vi "Try Match Response.vi"(8 "error in":errorcluster, 10 "ICAN CC Frame":refnum<class "ICAN CC Frame.lvclass">, 11 "Segmented Upload Transfer":refnum<class "Segmented Upload Transfer.lvclass">) -> (0 "error out":errorcluster, 2 "Match":bool, 3 "SDO Transfer":refnum<class "SDO Transfer.lvclass">)   [LabVIEW 2020, in "CANopen.lvlib" / "SDO Manager.lvlib" / "Segmented Upload Transfer.lvclass"]
uses:
  Segmented Upload Transfer.lvclass
  SDO Transfer/SDO Transfer.lvclass
  HAL/Source/Interfaces/ICAN CC Frame/ICAN CC Frame.lvclass
  Segmented Upload Transfer.lvclass/Segmented Upload Transfer.ctl
  CANopen Message/CANopen Message.lvclass
  SDO Transfer/SDO abort code.ctl
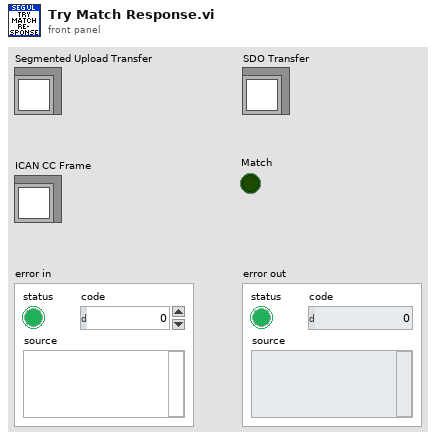
[diagram p1: front panel]
types:
  T1 = typedef "CANopen.lvlib/SDO Manager.lvlib/SDO Transfer.lvclass/SDO abort code.ctl" = u32
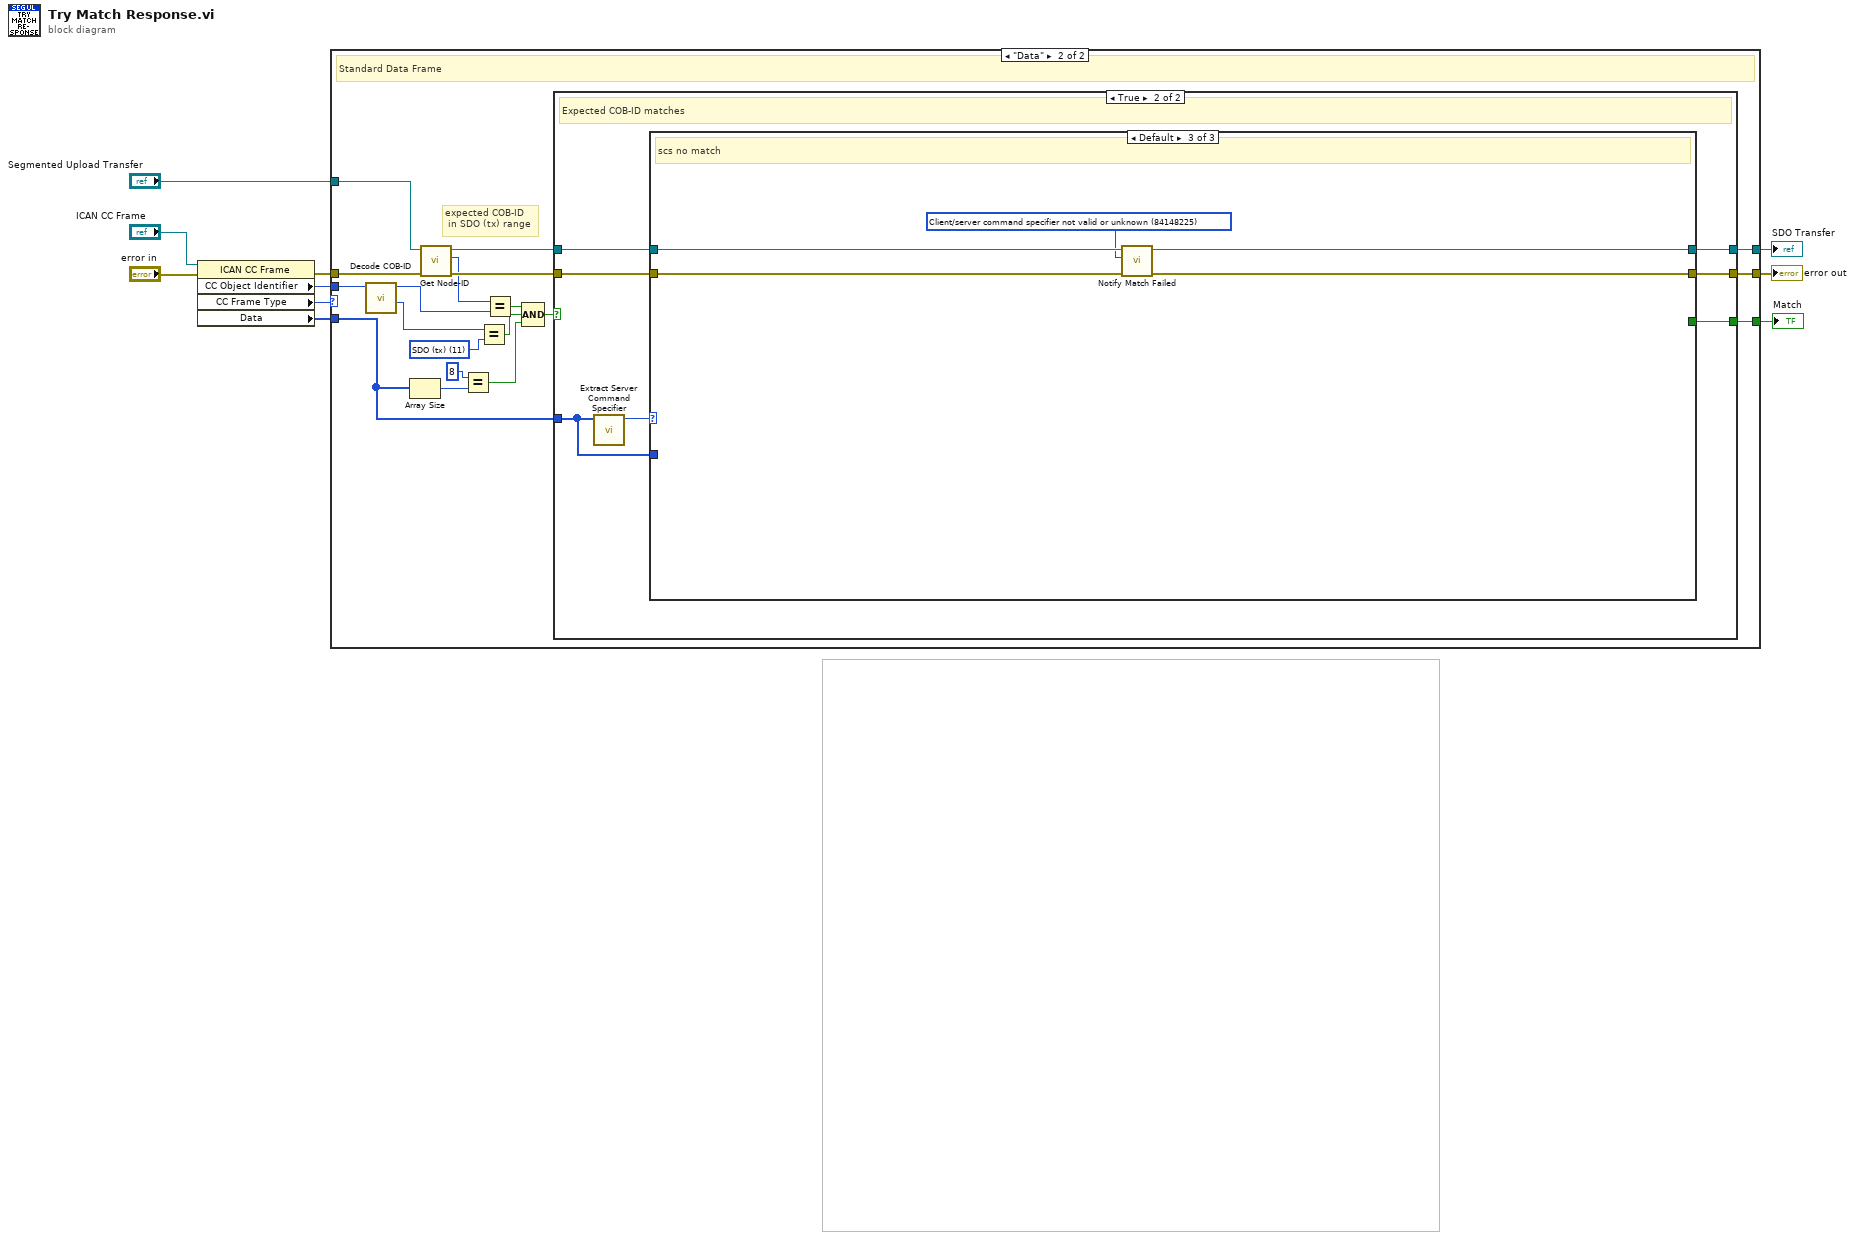
[diagram p0: block diagram]
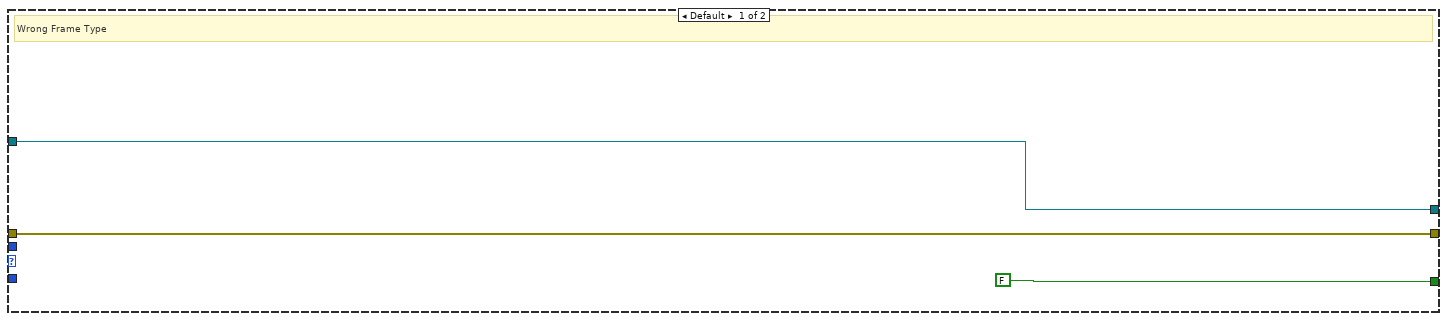
[diagram p2: hidden frame]
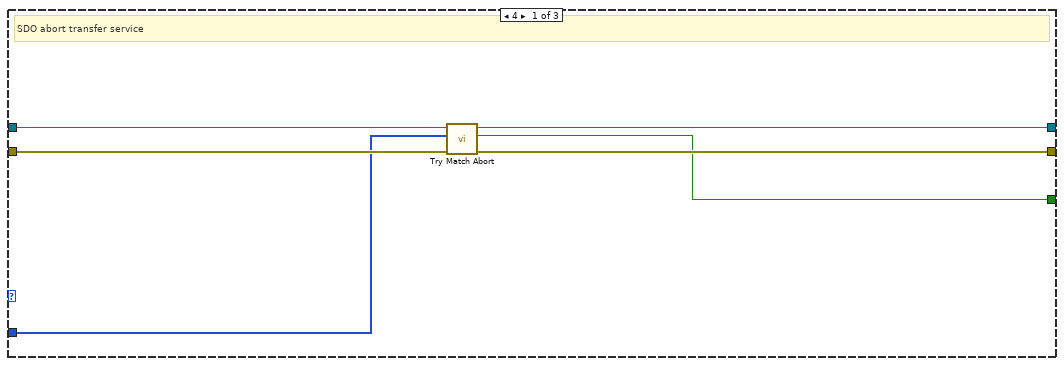
[diagram p4: hidden frame]
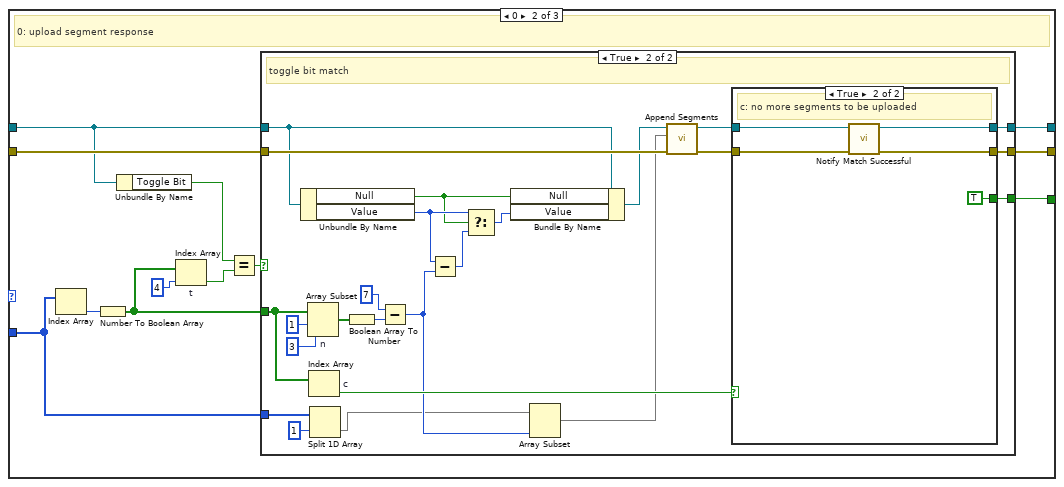
[diagram p5: hidden frame]
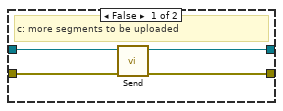
[diagram p7: hidden frame]
diagram:
  n1 = property class="ICAN CC Frame"(reference="ICAN CC Frame", error in="error in") -> (error out=w8:errorcluster, "CC Object Identifier"=w3:u32, "CC Frame Type"=w1:enum8{"Data", "Remote", "Error", "Overload"}, "Data"=w2:u8[])  [unwired: 1 out]
  n2 = case shown="\"Data\"" w1 {
    tunnel: w8 -> [w12 w32]
    tunnel: "Segmented Upload Transfer" -> [w11 w31]
    tunnel: [w11 w28] -> w6
    tunnel: [w12 w27] -> w5
    tunnel: [FALSE w26] -> w4
    tunnel: w3 -> [_ w25]
    tunnel: w2 -> [_ w14]
    frame Default {
      # "Wrong Frame Type"
    }
    frame "Data" {
      w22 = u8 11 items=["NMT"=0, "EMCY/SYNC"=1, "TIME"=2, "PDO1 (tx)"=3, "PDO1 (rx)"=4, "PDO2 (tx)"=5, "PDO2 (rx)"=6, "PDO3 (tx)"=7, "PDO3 (rx)"=8, "PDO4 (tx)"=9, "PDO4 (rx)"=10, "SDO (tx)"=11, "SDO (rx)"=12, "NMT error control"=14] ("Function Code")
      # "expected COB-ID\n in SDO (tx) range"
      # "Standard Data Frame"
      n3 = call "Decode COB-ID.vi"("COD-ID"=w25) -> ("Function Code"=w21:u8, "Node-ID"=w24:u8)  [unwired: 9 in]
      n4 = Array Size(array=w14) -> (size(s)=w20:i32)
      n5 = call "Get Node-ID.vi"("error in"=w32, "SDO Transfer in"=w31) -> ("error out"=w29:errorcluster, "Node-ID"=w23:u8, "SDO Transfer out"=w30:refnum<class "Segmented Upload Transfer.lvclass">)  [unwired: 7 in]
      n6 = Equal?(x=8, y=w20) -> (x = y?=w15:bool)
      n7 = Equal?(x=w21, y=w22) -> (x = y?=w16:bool)
      n8 = Equal?(x=w23, y=w24) -> (x = y?=w17:bool)
      n9 = Compound Arithmetic op=AND(w17, w16, w15) -> (w18:bool)
      n10 = case shown="True" w18 {
        tunnel: w30 -> [w34 w41]
        tunnel: w29 -> [w33 w40]
        tunnel: [w34 w38] -> w28
        tunnel: [w33 w39] -> w27
        tunnel: w14 -> [_ w35]
        tunnel: [_ w37] -> w26
        frame False {
          # "no match"
        }
        frame True {
          # "Expected COB-ID matches"
          n11 = call "Extract Server Command Specifier.vi"("Data"=w35) -> ("Server Command Specifier"=w36:u8)  [unwired: 10 in]
          n12 = case shown="Default" w36 {
            tunnel: w41 -> [w46 w55 w97]
            tunnel: w40 -> [w47 w59 w99]
            tunnel: [w45 w57 w96] -> w38
            tunnel: [w44 w58 w98] -> w39
            tunnel: [w43 w56 _] -> w37
            tunnel: w35 -> [w42 w49 _]
            frame 4 {
              # "SDO abort transfer service"
              n13 = call "Try Match Abort.vi"("error in"=w47, "Frame Data"=w42, "SDO Transfer in"=w46) -> ("error out"=w44:errorcluster, "Match"=w43:bool, "SDO Transfer out"=w45:refnum<class "Segmented Upload Transfer.lvclass">)  [unwired: 6 in]
            }
            frame 0 {
              # "0: upload segment response"
              n14 = Index Array(array=w49) -> (element=w48:u8)  [unwired: 1 in]
              n15 = Number To Boolean Array(number=w48) -> (Boolean array=w50:bool[])
              n16 = Unbundle By Name(w55) -> ("Toggle Bit"=w54:bool)
              n17 = Index Array "t"(array=w50, index=4 ("t")) -> (element=w51:bool)
              n18 = Equal?(x=w54, y=w51) -> (x = y?=w53:bool)
              n19 = case shown="True" w53 {
                tunnel: w59 -> [w60 w85]
                tunnel: [w60 w84] -> w58
                tunnel: [w61 w83] -> w57
                tunnel: [_ w82] -> w56
                tunnel: w55 -> [w61 w81]
                tunnel: w50 -> [_ w71]
                tunnel: w49 -> [_ w63]
                frame False {
                  # "#todo: sdo abort on toggle bit mismatch or just do nothing?"
                  # "toggle bit mismatch"
                }
                frame True {
                  # "toggle bit match"
                  n20 = Unbundle By Name(w81) -> ("Null"=w77:bool, "Value"=w80:u32)
                  n21 = Array Subset "n"(array=w71, index=1 ("n"), length=3) -> (w75:bool[])
                  n22 = Index Array "c"(array=w71) -> (element=w76:bool)  [unwired: 1 in]
                  n23 = Split 1D Array(array=w63, index=1) -> (second subarray=w62:u8[])  [unwired: 1 out]
                  n24 = Boolean Array To Number(Boolean array=w75) -> (number=w72:u32)
                  n25 = Subtract(x=u32 7, y=w72) -> (x-y=w65:u32)
                  n26 = Subtract(x=w80, y=w65) -> (x-y=w79:u32)
                  n27 = Select(t=w80, s=w77, f=w79) -> (s? t:f=w78:u32)
                  n28 = Bundle By Name(cluster=w81, "Null"=w77, "Value"=w78) -> (w68:refnum<class "Segmented Upload Transfer.lvclass">)
                  n29 = Array Subset(array=w62, length=w65) -> (w66:u8[])  [unwired: 1 in]
                  n30 = call "Append Segments.vi"("error in"=w85, "Segments"=w66, "Segmented Upload Transfer in"=w68) -> ("error out"=w69:errorcluster, "Segmented Upload Transfer out"=w67:refnum<class "Segmented Upload Transfer.lvclass">)  [unwired: 7 in]
                  n31 = case shown="True" w76 {
                    tunnel: w69 -> [w88 w93]
                    tunnel: [w87 w92] -> w84
                    tunnel: [w89 w90] -> w83
                    tunnel: [_ TRUE] -> w82
                    tunnel: w67 -> [w86 w91]
                    frame False {
                      # "c: more segments to be uploaded"
                      n32 = call-dynamic "Send.vi"("error in"=w88, "Segmented Upload Transfer"=w86) -> ("error out"=w87:errorcluster, "Segmented Upload Transfer"=w89:refnum<class "Segmented Upload Transfer.lvclass">)  [unwired: 8 in]
                    }
                    frame True {
                      # "c: no more segments to be uploaded"
                      n33 = call "Notify Match Successful.vi"("error in"=w93, "SDO Transfer in"=w91) -> ("error out"=w92:errorcluster, "SDO Transfer out"=w90:refnum<class "Segmented Upload Transfer.lvclass">)  [unwired: 8 in]
                    }
                  }
                }
              }
            }
            frame Default {
              w95 = T1 84148225 items=["Toggle bit not allowed"=84082688, "SDO protocol timed out"=84148224, "Client/server command specifier not valid or unknown"=84148225, "Invalid block size (block mode only)"=84148226, "Invalid sequence number (block mode only)"=84148227, "CRC error (block mode only)"=84148228, "Out of memory"=84148229, "Attempt to read a write only object"=100728833, "Attempt to write a read only object"=100728834, "Object does not exist in the object dictionary"=100794368, "Object cannot be mapped to the PDO"=100925505, "The number and length of the objects to be mapped would exceed PDO length"=100925506, "General parameter incompatibility reason"=100925507, "General internal incompatibility in the device"=100925511, "Access failed due to an hardware error"=101056512, "Data type does not match, length of service parameter does not match"=101122064, "Data type does not match, length of service parameter too high"=101122066, "Data type does not match, length of service parameter too low"=101122067, "Sub-index does not exist"=101253137, "Invalid value for parameter (download only)"=101253168, "Value of parameter written too high (download only)"=101253169, "Value of parameter written too low (download only)"=101253170, "Maximum value is less than minimum value"=101253174, "Resource not available: SDO connection"=101318691, "General error"=134217728, "Data cannot be transferred or stored to the application"=134217760, "Data cannot be transferred or stored to the application because of local control"=134217761, "Data cannot be transferred or stored to the application because of the present device stable"=134217762, "Object dictionary dynamic generation fails or no object dictionary is present (e.g. object dictionary is generated from file and generation fails because of an file error)"=134217763, "No data available"=134217764] ("SDO abort code")
              # "scs no match"
              n34 = call "Notify Match Failed.vi"("error in"=w99, "SDO abort code"=w95, "SDO Transfer in"=w97) -> ("error out"=w98:errorcluster, "SDO Transfer out"=w96:refnum<class "Segmented Upload Transfer.lvclass">)  [unwired: 7 in]
            }
          }
        }
      }
    }
  }
  "SDO Transfer" <- w6
  "error out" <- w5
  "Match" <- w4
